vi "Unpause Front Panel Updates.vi"(8 "error in (no error)":errorcluster, 11 "CIF_UI in":refnum<class "CIF_UI.lvclass">) -> (0 "error out":errorcluster, 3 "CIF_UI out":refnum<class "CIF_UI.lvclass">)   [LabVIEW 2021, in "CIF_UI.lvclass"]
uses:
  CIF_UI.lvclass
  CIF_UI.lvclass/CIF_UI.ctl
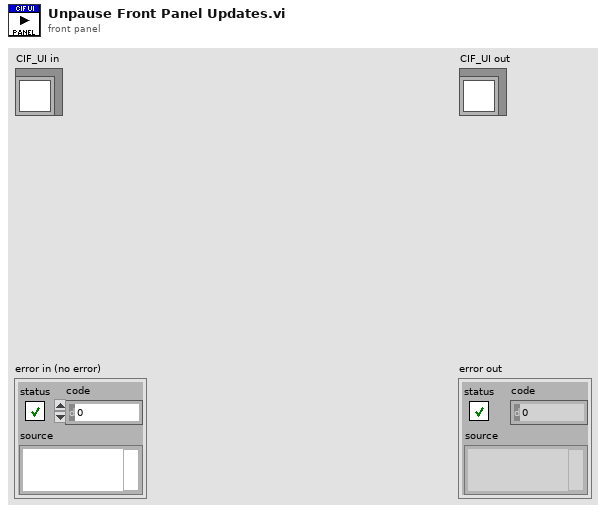
[diagram p1: front panel]
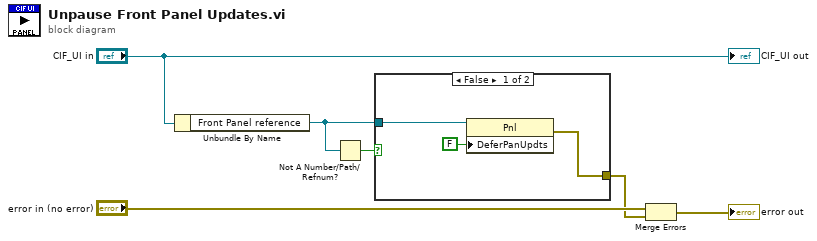
[diagram p0: block diagram]
diagram:
  n1 = Unbundle By Name("CIF_UI in") -> ("Front Panel reference"=w5:refnum<vi>)
  n2 = Not A Number/Path/Refnum?(number/path/refnum=w5) -> (NaN/Path/Refnum?=w4:bool)
  n3 = case shown="False" w4 {
    tunnel: w5 -> [w8 _]
    tunnel: [w7 _] -> w2
    frame False {
      n4 = property class="Pnl"(reference=w8, "DeferPanUpdts"=FALSE ("Defer Panel Updates")) -> (error out=w7:errorcluster)  [unwired: 1 in, 1 out]
    }
    frame True {
      # "FP Reference is not valid"
    }
  }
  n5 = Merge Errors("error in (no error)", w2) -> (→"error out":errorcluster)
  "CIF_UI out" <- "CIF_UI in"
